vi "SEQ Start sequence.vi"(8 "error in (no error)":errorcluster, 10 "sequence.cont":bool, 11 "Refnum in":T1) -> (0 "error out":errorcluster, 3 "Refnum out":T1)   [LabVIEW 2019, in "FPGA sequencer API.lvlib"]
uses:
  FPGA sequencer API.lvlib
  FPGA sequencer ref.ctl
  5fcfb919-2c82-4480-bc80-027d0fe5dd30.vi
  <vilib>/Utility/error.llb/Error Cluster From Error Code.vi
  <vilib>/rvi/errors/niLvFpgaAdjustHostInterfaceError.vi
  <vilib>/rvi/interface/nirviReadWriteControl/nirviReadWriteControl.xnode
  NiFpgaLv.dll
  <vilib>/rvi/interface/Simulation/niFpgaSimulationCallBeginRW.vi
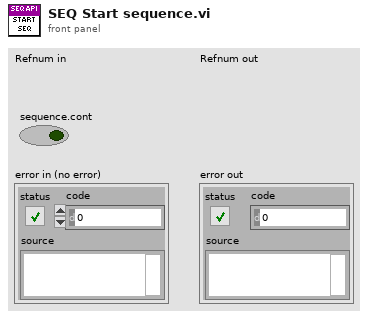
[diagram p1: front panel]
types:
  T1 = typedef "FPGA sequencer API.lvlib/FPGA sequencer ref.ctl" = refnum<k20>
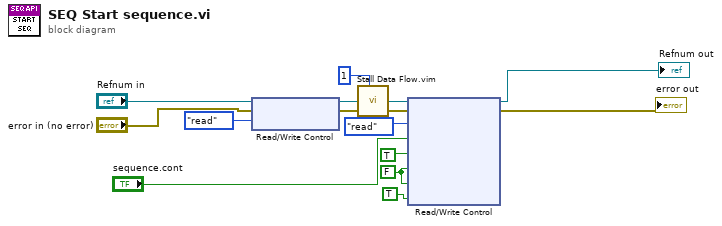
[diagram p0: block diagram]
diagram:
  w2 = FALSE ("seq.start")
  n1 = xnode "Read/Write Control"("FPGA VI Reference In"="Refnum in", "error in"="error in (no error)", "memo mode"=enum16{"flush", "reset", "write", "read"}."read" ("dram mode")) -> ("FPGA VI Reference Out"=w6:T1, "error out"=w5:errorcluster)
  n2 = call "Stall Data Flow.vim"("value in"=w6, "milliseconds to wait"=u32 1) -> ("value out"=w4:T1)  [unwired: 1 out]
  n3 = xnode "Read/Write Control"("FPGA VI Reference In"=w4, "error in"=w5, "memo mode"=enum16{"flush", "reset", "write", "read"}."read" ("dram mode"), "seq.continous"="sequence.cont", "seq.start"=TRUE, "seq.rst"=w2, "seq.start"=w2, "gen.enable"=TRUE ("seq.start")) -> ("FPGA VI Reference Out"=→"Refnum out":T1, "error out"=→"error out":errorcluster)
